vi "Close.vi"(8 "error in (no error)":errorcluster, 10 "Reason":T1, 11 "Panel in":refnum<class "Panel.lvclass">) -> (0 "error out":errorcluster, 3 "Panel out":refnum<class "Panel.lvclass">)   [LabVIEW 2014, in "OOPanel.lvlib" / "Panel.lvclass"]
uses:
  Panel.lvclass
  Close Reason.ctl
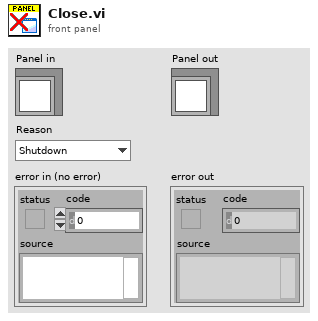
[diagram p1: front panel]
types:
  T1 = typedef "OOPanel.lvlib/Panel.lvclass/Close Reason.ctl" = enum16{"Shutdown", "Close"}
  T2 = typedef "OOPanel.lvlib/Panel.lvclass/Ref Data.ctl" = cluster{"Panel Events":T3, "Panel Ref":refnum<vi>, "SubPanel":refnum<vi>, "Close":bool, "Running":bool, "State":T4}
  T3 = typedef "OOPanel.lvlib/Panel.lvclass/Panel Events.ctl" = cluster{"Visbility":refnum<user-event>, "Close":refnum<user-event>}
  T4 = typedef "OOPanel.lvlib/Panel.lvclass/Visibility State.ctl" = enum16{"Idle", "Closed", "Hidden", "Visible", "Subpanel"}
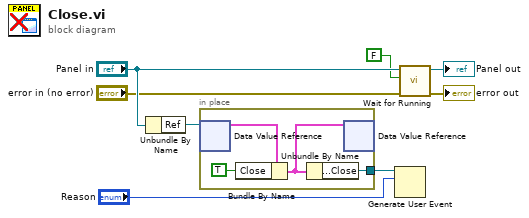
[diagram p0: block diagram]
diagram:
  n1 = Unbundle By Name("Panel in") -> ("Ref"=w8:refnum<data-value>)
  n2 = in-place {
    in-place-border: [w9] -> w7
    n3 = in-place-dvr #1(w8) -> (w12:T2)  [unwired: 1 out]
    n4 = Bundle By Name(cluster=w12, "Close"=TRUE) -> (w10:T2)
    n5 = Unbundle By Name(w10) -> ("Panel Events.Close"=w9:refnum<user-event>)
    n6 = in-place-dvr #1(w10) -> ()  [unwired: 2 out]
  }
  n7 = Generate User Event(user event=w7, event data cluster="Reason") -> ()  [unwired: 2 in, 2 out]
  n8 = call "Wait for Running.vi"("error in (no error)"="error in (no error)", "Running"=FALSE, "Panel in"="Panel in") -> ("error out"=→"error out":errorcluster, "Panel out"=→"Panel out":refnum<class "Panel.lvclass">)  [unwired: 7 in]
